vi "OEE_SCREEN_2_show_label_for_graphics_acc.vi"(10 "Y_annotation_offset":dbl, 11 "values":cluster{dbl[], dbl[]}) -> (3 "Array":T1(array[cluster]))   [LabVIEW 2020]
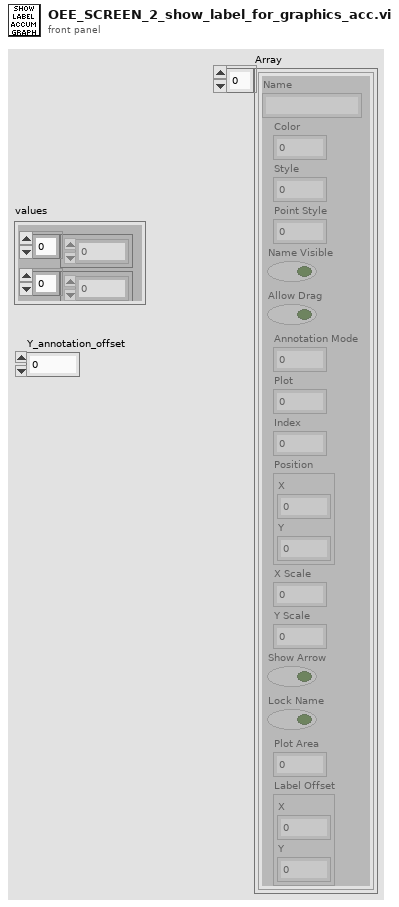
[diagram p1: front panel]
types:
  T1 = cluster{"Name":string, "Color":u32, "Style":u8, "Point Style":u8, "Name Visible":bool, "Allow Drag":bool, "Annotation Mode":u32, "Plot":i32, "Index":i32, "Position":cluster{"X":dbl, "Y":dbl}, "X Scale":u32, "Y Scale":u32, "Show Arrow":bool, "Lock Name":bool, "Plot Area":i32, "Label Offset":cluster{"X":dbl, "Y":dbl}}[]
  T2 = cluster{"Name":string, "Color":u32, "Style":u8, "Point Style":u8, "Name Visible":bool, "Allow Drag":bool, "Annotation Mode":u32, "Plot":i32, "Index":i32, "Position":cluster{"X":dbl, "Y":dbl}, "X Scale":u32, "Y Scale":u32, "Show Arrow":bool, "Lock Name":bool, "Plot Area":i32, "Label Offset":cluster{"X":dbl, "Y":dbl}}
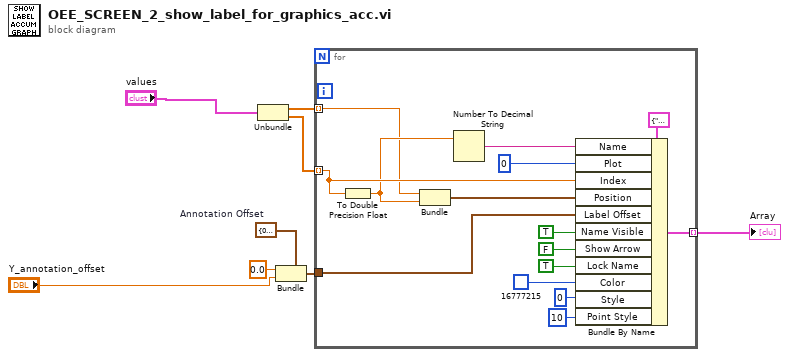
[diagram p0: block diagram]
diagram:
  w6 = cluster{dbl, dbl} {0.0, 0.0}  # Annotation Offset
  n1 = Unbundle("values") -> (w4:dbl[], w5:dbl[])
  n2 = Bundle(cluster=w6, 0.0, "Y_annotation_offset") -> (w7:cluster{dbl, dbl})
  n3 = for {
    tunnel: w5 -> [w16] mode=indexing
    tunnel: [w18] -> w3 mode=indexing
    tunnel: w4 -> [w11] mode=indexing
    tunnel: w7 -> [w9]
    n4 = To Double Precision Float(number=w16) -> (double precision float=w12:dbl)
    n5 = Bundle(w11, w12) -> (w13:cluster{dbl, dbl})  [unwired: 1 in]
    n6 = Number To Decimal String(number=w12) -> (decimal integer string=w22:string)  [unwired: 1 in]
    n7 = Bundle By Name(cluster=T2 {"Name"="", "Color"=0, "Style"=0, "Point Style"=0, "Name Visible"=FALSE, "Allow Drag"=FALSE, "Annotation Mode"=0, "Plot"=0, "Index"=0, "Position"={"X"=0.0, "Y"=0.0}, "X Scale"=0, "Y Scale"=0, "Show Arrow"=FALSE, "Lock Name"=FALSE, "Plot Area"=0, "Label Offset"={"X"=0.0, "Y"=0.0}}, "Name"=w22, "Plot"=0, "Index"=w16, "Position"=w13, "Label Offset"=w9, "Name Visible"=TRUE, "Show Arrow"=FALSE, "Lock Name"=TRUE, "Color"=u32 16777215, "Style"=u8 0, "Point Style"=u8 10) -> (w18:T2)
  }
  "Array" <- w3
